vi "POLL BIAS.vi"(8 "error in (no error)":errorcluster, 9 "element":T1 {"Avoid zero threshold (V)" format="%#_13g"}, 10 "ScanQ in":refnum<queue>, 11 "Queue in":refnum<queue>) -> (0 "error out":errorcluster, 2 "ScanQ out":refnum<queue>, 3 "Queue out":refnum<queue>)   [LabVIEW 2025]
uses:
  <userlib>/Nanonis Prog Interface V5e/Nanonis Prog Interface.lvlib
  Labview-File/STM-Auto-Project Testing/STM-Auto-Project (Trial 2)/QMH CTLS/Scan_Params (QMH).ctl
  TEMP_SWEEPER.ctl
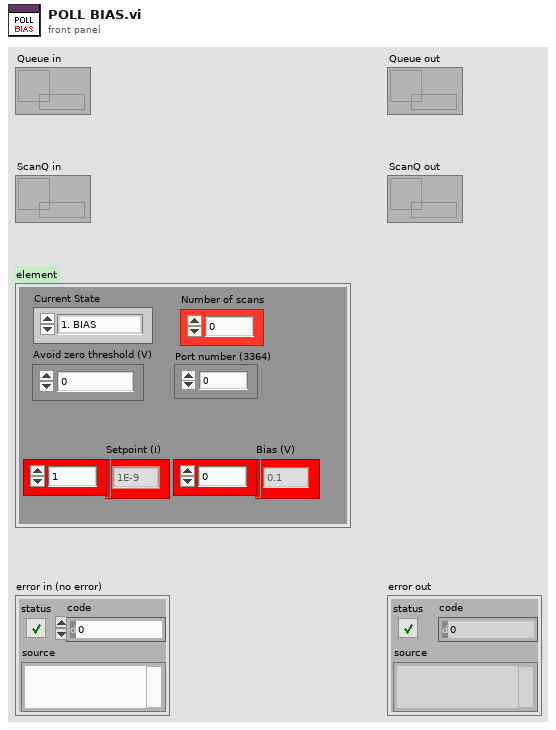
[diagram p1: front panel]
types:
  T1 = typedef "Scan_Params (QMH).ctl" = cluster{"Setpoint (I)":dbl[], "Bias (V)":dbl[], "Number of scans":u8, "Port number (3364)":u32, "Avoid zero threshold (V)":dbl, "Current State":enum16{"1. BIAS", "2. INIT_SCAN", "3. SCAN_IDLE", "4. INTER_SCAN", "5. NEW_COORDS_&_FRAME", "6. FINAL_SCAN", "7. STOP"}}
  T2 = enum16{"1. BIAS", "2. INIT_SCAN", "3. SCAN_IDLE", "4. INTER_SCAN", "5. NEW_COORDS_&_FRAME", "6. FINAL_SCAN", "7. POLL_BIAS", "8. Z-CONT.", "9. STOP"}
  T3 = enum16{"SET TEMP", "SWEEP IDLE", "NEXT TEMP", "SWEEP DONE"}
  T4 = typedef "TEMP_SWEEPER.ctl" = cluster{"Temps(K)":dbl[], "Sweep States":enum16{"SET TEMP", "SWEEP IDLE", "NEXT TEMP", "SWEEP DONE"}}
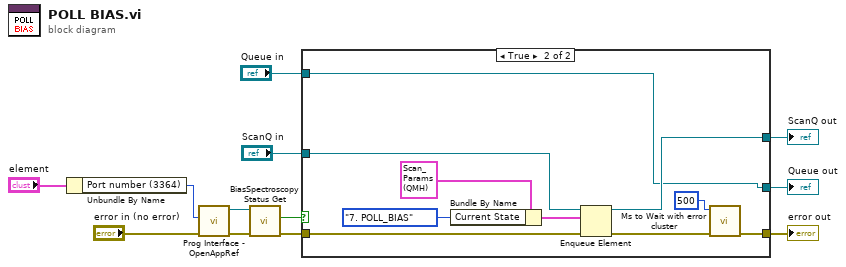
[diagram p0: block diagram]
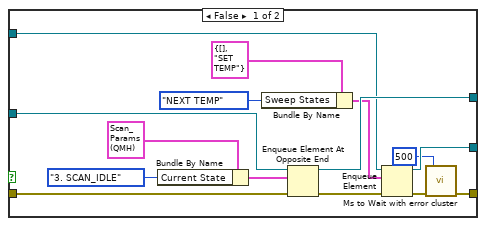
[diagram p2: hidden frame]
diagram:
  n1 = Unbundle By Name("element") -> ("Port number (3364)"=w1:u32)
  n2 = call <userlib>:"Prog Interface - OpenAppRef.vi"("Error in (no error)"="error in (no error)", "Port number (3364)"=w1) -> ("Error out"=w4:errorcluster, "Application reference"=w3:refnum<vi>)  [unwired: 4 in]
  n3 = call <userlib>:"BiasSpectroscopy Status Get.vi"("Error in (no error)"=w4, "Application ref in"=w3) -> ("Error out"=w11:errorcluster, "Running?"=w5:bool)  [unwired: 5 in, 1 out]
  n4 = case shown="True" w5 {
    tunnel: "ScanQ in" -> [w27 w37]
    tunnel: [w24 w34] -> w7
    tunnel: "Queue in" -> [w23 w32]
    tunnel: [w22 w32] -> w9
    tunnel: [w14 w29] -> w10
    tunnel: w11 -> [w18 w33]
    frame False {
      n5 = Bundle By Name(cluster=T1 {"Setpoint (I)"=[], "Bias (V)"=[], "Number of scans"=1, "Port number (3364)"=3364, "Avoid zero threshold (V)"=0.004999999888241291, "Current State"=enum."1. BIAS"} ("element"), "Current State"=T2."3. SCAN_IDLE") -> (w25:T1)
      n6 = Bundle By Name(cluster=T4 {"Temps(K)"=[], "Sweep States"=enum."SET TEMP"} ("Temp and Field Range"), "Sweep States"=T3."NEXT TEMP") -> (w20:T4)
      n7 = Enqueue Element At Opposite End(queue=w27, element=w25, error in (no error)=w18) -> (queue out=w24:refnum<queue>, error out=w19:errorcluster)  [unwired: 1 in, 1 out]
      n8 = Enqueue Element(queue=w23, element=w20, error in (no error)=w19) -> (queue out=w22:refnum<queue>, error out=w15:errorcluster)  [unwired: 1 in, 1 out]
      n9 = call <userlib>:"Ms to Wait with error cluster.vi"("error in (no error)"=w15, "milliseconds to wait"=u32 500) -> ("error out"=w14:errorcluster)  [unwired: 4 in, 1 out]
    }
    frame True {
      n10 = Bundle By Name(cluster=T1 {"Setpoint (I)"=[], "Bias (V)"=[], "Number of scans"=1, "Port number (3364)"=3364, "Avoid zero threshold (V)"=0.004999999888241291, "Current State"=enum."1. BIAS"} ("element"), "Current State"=T2."7. POLL_BIAS") -> (w35:T1)
      n11 = Enqueue Element(queue=w37, element=w35, error in (no error)=w33) -> (queue out=w34:refnum<queue>, error out=w30:errorcluster)  [unwired: 1 in, 1 out]
      n12 = call <userlib>:"Ms to Wait with error cluster.vi"("error in (no error)"=w30, "milliseconds to wait"=u32 500) -> ("error out"=w29:errorcluster)  [unwired: 4 in, 1 out]
    }
  }
  "error out" <- w10
  "Queue out" <- w9
  "ScanQ out" <- w7
